vi "calculate.vi"(8 "error in (no error)":errorcluster, 10 "Numbers.lvclass":refnum<class "Numbers.lvclass">, 11 "Subtract in":refnum<class "Subtract.lvclass">) -> (0 "error out":errorcluster, 3 "Subtract out":refnum<class "Subtract.lvclass">)   [LabVIEW 2017, in "Subtract.lvclass"]
uses:
  Subtract.lvclass
  Numbers Class/Numbers.lvclass
  Numbers Class/Numbers.lvclass/Numbers.ctl
  Subtract.lvclass/Subtract.ctl
  Chain Class/Chain.lvclass
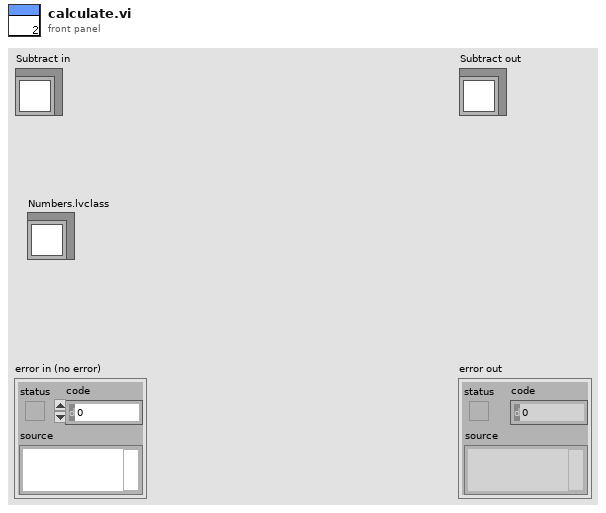
[diagram p1: front panel]
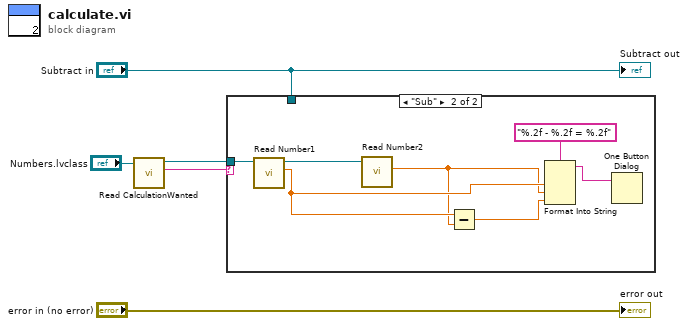
[diagram p0: block diagram]
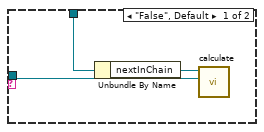
[diagram p2: hidden frame]
diagram:
  n1 = call "Read CalculationWanted.vi"("Numbers in"="Numbers.lvclass") -> ("CalculationWanted"=w3:string, "Numbers out"=w4:refnum<class "Numbers.lvclass">)  [unwired: 8 in, 1 out]
  n2 = case shown="\"Sub\"" w3 {
    tunnel: w4 -> [w8 w15]
    tunnel: "Subtract in" -> [w7 _]
    frame "False", Default {
      n3 = Unbundle By Name(w7) -> ("nextInChain"=w6:refnum<class "Chain.lvclass">)
      n4 = call-dynamic "calculate.vi"("Numbers.lvclass"=w8, "Chain in"=w6) -> ()  [unwired: 8 in, 2 out]
    }
    frame "Sub" {
      n5 = call "Read Number1.vi"("Numbers in"=w15) -> ("Number1"=w10:dbl, "Numbers out"=w14:refnum<class "Numbers.lvclass">)  [unwired: 8 in, 1 out]
      n6 = call "Read Number2.vi"("Numbers in"=w14) -> ("Number2"=w9:dbl)  [unwired: 8 in, 2 out]
      n7 = Subtract(x=w10, y=w9) -> (x-y=w12:dbl)
      n8 = Format Into String(format string="%.2f - %.2f = %.2f", w10, w9, w12) -> (resulting string=w11:string)  [unwired: 2 in, 1 out]
      n9 = One Button Dialog(message=w11) -> ()  [unwired: 1 in, 1 out]
    }
  }
  "error out" <- "error in (no error)"
  "Subtract out" <- "Subtract in"
